vi "write_params.vi"(8 "error in (no error)":errorcluster, 10 "params":T1={"nu"=0.5, "C"=1.0, "kernel"="rbf", "degree"=3.0, "gamma"={"gamma_type"="scale", "gamma_float"=0.001}, "coef0"=0.0, "shrinking"=TRUE, "tol"=0.001, "cache_size"=200.0, "verbose"=FALSE, "max_iter"=-1.0}, 11 "NuSVR in":refnum<class "NuSVR.lvclass">) -> (0 "error out":errorcluster, 3 "NuSVR out":refnum<class "NuSVR.lvclass">)   [LabVIEW 2020, in "NuSVR.lvclass"]
uses:
  NuSVR.lvclass
  Controls/nu_svr_params.ctl
  NuSVR.lvclass/NuSVR.ctl
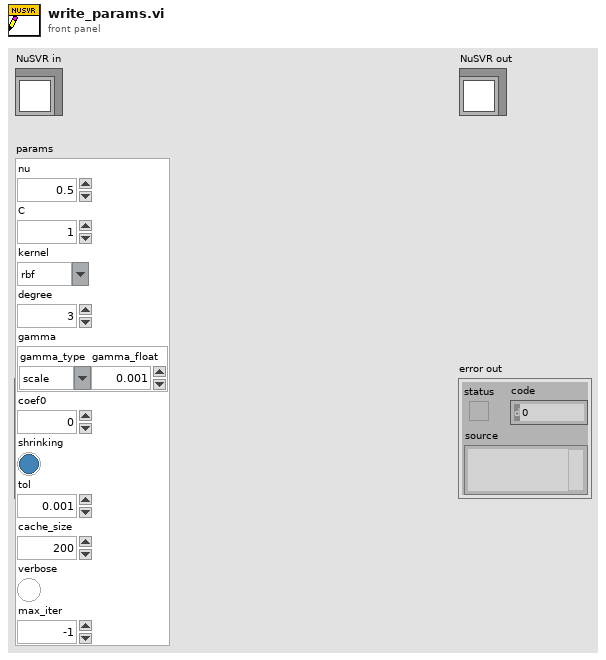
[diagram p1: front panel]
types:
  T1 = typedef "nu_svr_params.ctl" = cluster{"nu":dbl, "C":dbl, "kernel":string, "degree":dbl, "gamma":cluster{"gamma_type":string, "gamma_float":dbl}, "coef0":dbl, "shrinking":bool, "tol":dbl, "cache_size":dbl, "verbose":bool, "max_iter":dbl}
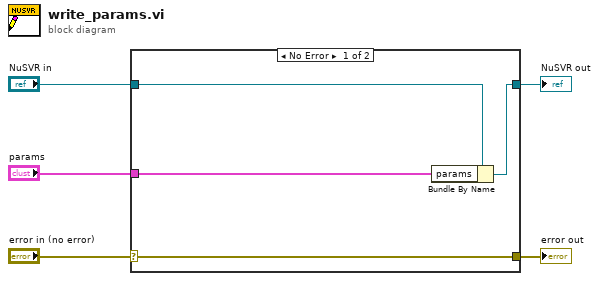
[diagram p0: block diagram]
diagram:
  n1 = case shown="No Error" "error in (no error)" {
    selector: "error in (no error)" -> [w9 w10]
    tunnel: [w9 w10] -> w4
    tunnel: [w7 w11] -> w2
    tunnel: "NuSVR in" -> [w8 w11]
    tunnel: "params" -> [w6 _]
    frame No Error {
      n2 = Bundle By Name(cluster=w8, "params"=w6) -> (w7:refnum<class "NuSVR.lvclass">)
    }
    frame Error {
    }
  }
  "error out" <- w4
  "NuSVR out" <- w2
